vi "ConnectionData.vi"(1 "AxisNo":u16) -> (0 "ConnectionDataOUT":T1={"DeviceIDCtrl"=1, "ProtocolCtrl"=enum."Modbus RTU", "COMportCtrl"="COM2", "IPCtrl"="", "serial master instance"=refnum, "ConnectionStatusIndicator"=FALSE})   [LabVIEW 2020, in "SMCD14_lib.lvlib"]
uses:
  ConnectionData_typedef.ctl
  <vilib>/Modbus/master/Modbus Master.lvclass
  Globals.vi
  SMCD14_lib.lvlib
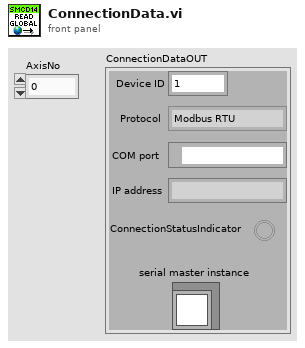
[diagram p1: front panel]
types:
  T1 = typedef "SMCD14_lib.lvlib/ConnectionData_typedef.ctl" = cluster{"DeviceIDCtrl":u16, "ProtocolCtrl":enum16{"Modbus RTU", "Modbus TCP", ""}, "COMportCtrl":refnum<visa-resource-name>, "IPCtrl":string, "serial master instance":refnum<class "Modbus Master.lvclass">, "ConnectionStatusIndicator":bool}
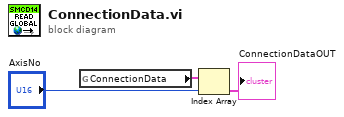
[diagram p0: block diagram]
diagram:
  n1 = global read "Globals.vi" "ConnectionData"() -> (w2:T1[])
  n2 = Index Array(array=w2, index="AxisNo") -> (element=→"ConnectionDataOUT":T1)
